vi "子界面-评定报告生成.vi"(1 "反射图路径":path, 5 "标注后的图片路径":path, 6 "总面积":i32, 7 "部位":string, 8 "穿透图路径":path, 9 "测试人":string, 10 "产品序号":string) -> (3 "写入数据库路径":path)   [LabVIEW 2018]
uses:
  <vilib>/Utility/NIReport.llb/Report Type.ctl
  <vilib>/addons/database/Connection.llb/DB Tools Open Connec (String).vi
  <vilib>/Utility/NIReport.llb/Append Report Text (str wrap).vi
  <vilib>/Utility/NIReport.llb/Append Report Text (num wrap).vi
  <vilib>/Utility/NIReport.llb/Append Image to Report (path wrap).vi
  <vilib>/addons/database/_DB Variant To Data/Database Variant To Data.xnode
  <vilib>/Utility/NIReport.llb/NI_report.lvclass
  <vilib>/addons/database/NI_Database_API.lvlib
  <vilib>/Utility/NIReport.llb/NI_ReportGenerationCore.lvlib
  <vilib>/Utility/NIReport.llb/Word/NI_Word.lvclass
panel:
  out "报告生成路径":path
  out "最大Z值":cluster{dbl}
  out "评定等级":string
  out "data":T1
  out "评定等级2":string caption="评定等级"
  out "缺陷占比(%)":dbl
  out "数值":dbl
  in  "返回 2":bool
  out "data 2":T1
  # "评定和分级结果"
  # "分层类"
  # "弥散类"
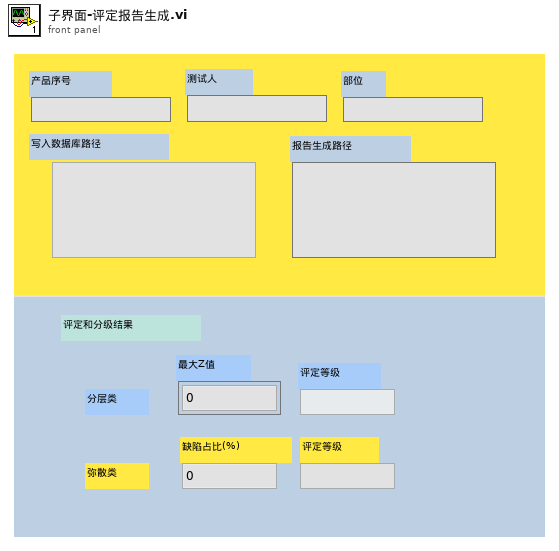
[diagram p1: front panel]
types:
  T1 = typedef "Z值ctl.ctl" = cluster{dbl}[]
  T2 = cluster{"position (excel)":cluster{"row":i32, "column":i32}, "name (excel)":string, "bookmark (word)":string}
  T3 = cluster{"position (Excel)":cluster{"row":i32, "column":i32}, "name (Excel)":string, "bookmark (Word)":string}
  T4 = typedef "NI_ReportGenerationCore.lvlib/Report Type.ctl" = enum16{"HTML", "Word", "Excel"}
  T5 = typedef "NI_Database_API.lvlib/Conn ObjectReference.ctl" = refnum<k1>
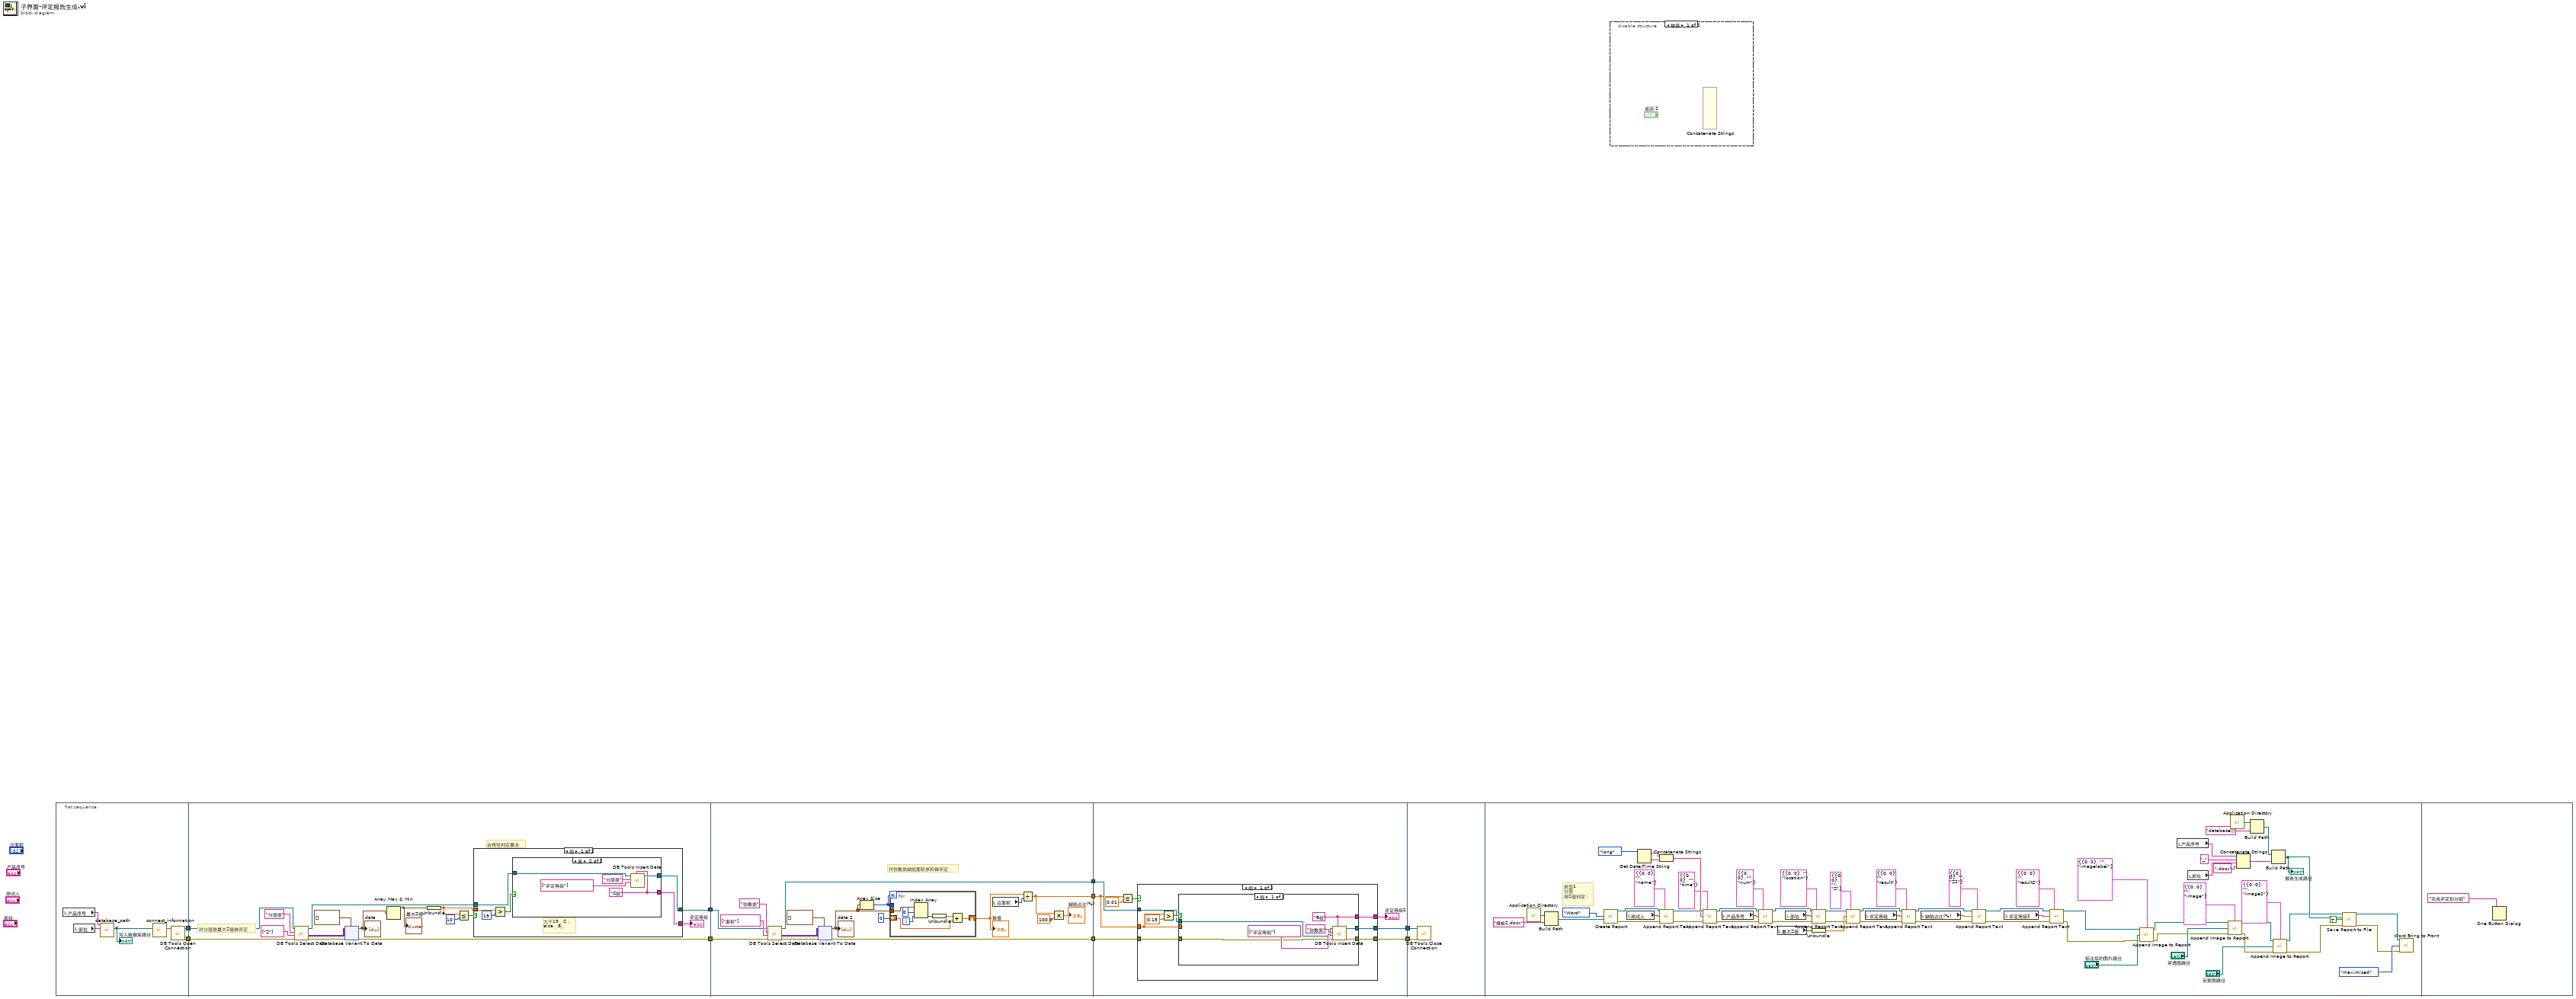
[diagram p0: block diagram]
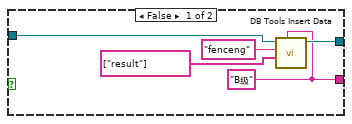
[diagram p2: hidden frame]
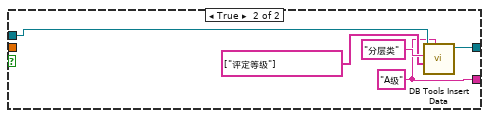
[diagram p3: hidden frame]
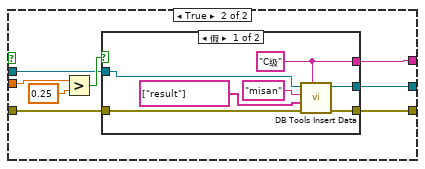
[diagram p4: hidden frame]
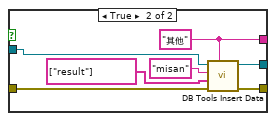
[diagram p5: hidden frame]
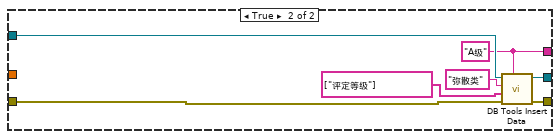
[diagram p6: hidden frame]
diagram:
  n1 = flat-sequence {
    tunnel: [w11] -> w9
    tunnel: [w10] -> w8
    tunnel: w9 -> [w25]
    tunnel: w8 -> [w28]
    tunnel: [w19] -> w7
    tunnel: [w17] -> w6
    tunnel: [w104] -> w5
    tunnel: w7 -> [w108]
    tunnel: w6 -> [w105]
    tunnel: [w103] -> w4
    tunnel: [w96] -> w3
    tunnel: w5 -> [w162]
    tunnel: w4 -> [w164]
    tunnel: [w163] -> w2
    tunnel: [w161] -> w1
    tunnel: w3 -> [w160]
    tunnel: w2 -> [w212]
    tunnel: w1 -> [w211]
    frame #0 {
      n2 = local read "产品序号"() -> (w13:string)
      n3 = local read "部位"() -> (w12:string)
      n4 = call "database_path.vi"("部位"=w12, "产品序号"=w13) -> ("database path"=w14:path)  [unwired: 9 in]
      "写入数据库路径" <- w14
      n5 = call "connect_information.vi"("路径"=w14) -> ("connect info"=w15:string)  [unwired: 10 in]
      n6 = call-poly <vilib>:"DB Tools Open Connection.vi"("connection information"=w15) -> ("error out"=w10:errorcluster, "connection reference"=w11:T5)  [unwired: 7 in]
    }
    frame #1 {
      # "合格性判定算法"
      # "对分层类最大Z值做评定"
      n7 = call <vilib>:"DB Tools Select Data.vi"("error in (no error)"=w28, "columns"=string[] ["Z"], "table"="分层类", "connection reference"=w25) -> ("error out"=w29:errorcluster, "data"=w27:variant[][], "connection reference out"=w20:T5)  [unwired: 2 in]
      n8 = xnode "Database Variant To Data"("database variant"=w27, "error in (no error)"=w29, "type"=T1 []) -> ("data"=w24:T1, "error out"=w17:errorcluster)
      "data" <- w24
      n9 = Array Max & Min(array=w24) -> (max value=w21:cluster{dbl})  [unwired: 3 out]
      "最大Z值" <- w21
      n10 = Unbundle(w21) -> (w18:dbl)
      n11 = Less Or Equal?(x=w18, y=10) -> (x <= y?=w22:bool)
      n12 = case shown="假" w22 {
        tunnel: w20 -> [w35 w52]
        tunnel: [w34 w49] -> w19
        tunnel: w18 -> [w33 _]
        tunnel: [w32 w48] -> w16
        frame False {
          # "大于19，C；\nelse，B。"
          n13 = Greater?(x=w33, y=19) -> (0:w36:bool)
          n14 = case shown="真" w36 {
            tunnel: w35 -> [w40 w44]
            tunnel: [w39 w45] -> w34
            tunnel: [w38 w43] -> w32
            frame False {
              w38 = "B级"
              n15 = call <vilib>:"DB Tools Insert Data.vi"("data"=w38, "columns"=string[] ["result"], "table"="fenceng", "connection reference"=w40) -> ("connection reference out"=w39:T5)  [unwired: 6 in, 1 out]
            }
            frame True {
              w43 = "C级"
              n16 = call <vilib>:"DB Tools Insert Data.vi"("data"=w43, "columns"=string[] ["评定等级"], "table"="分层类", "connection reference"=w44) -> ("connection reference out"=w45:T5)  [unwired: 6 in, 1 out]
            }
          }
        }
        frame True {
          w48 = "A级"
          n17 = call <vilib>:"DB Tools Insert Data.vi"("data"=w48, "columns"=string[] ["评定等级"], "table"="分层类", "connection reference"=w52) -> ("connection reference out"=w49:T5)  [unwired: 6 in, 1 out]
        }
      }
      "评定等级" <- w16
    }
    frame #2 {
      # "对弥散类缺陷面积求和做评定"
      n18 = call <vilib>:"DB Tools Select Data.vi"("error in (no error)"=w105, "columns"=string[] ["面积"], "table"="弥散类", "connection reference"=w108) -> ("error out"=w106:errorcluster, "data"=w107:variant[][], "connection reference out"=w103:T5)  [unwired: 2 in]
      n19 = xnode "Database Variant To Data"("database variant"=w107, "error in (no error)"=w106, "type"=T1 []) -> ("data"=w101:T1, "error out"=w104:errorcluster)
      "data 2" <- w101
      n20 = Array Size(array=w101) -> (size(s)=w100:i32)
      n21 = for {
        N: w100 -> [_]
        tunnel: w101 -> [w117]
        tunnel: w100 -> [_]
        shift-right: [w112] -> w98
        shift-left: 0 -> [w111]
        i -> [w115]
        n22 = Index Array(array=w117, index #1=0 ("索引 (列)"), index #2=w115) -> (element #2=w114:cluster{dbl})  [unwired: 1 out]
        n23 = Unbundle(w114) -> (w113:dbl)
        n24 = Add(x=w113, y=w111) -> (x+y=w112:dbl)
      }
      "数值" <- w98
      n25 = local read "总面积"() -> (w97:i32)
      n26 = Divide(x=w98, y=w97) -> (x/y=w96:dbl)
      n27 = Multiply(x=w96, y=100.0) -> (x*y=→"缺陷占比(%)":dbl)
    }
    frame #3 {
      n28 = Less Or Equal?(x=w160, y=0.01) -> (x <= y?=w166:bool)
      n29 = case shown="假" w166 {
        tunnel: w164 -> [w171 w208]
        tunnel: [w170 w207] -> w163
        tunnel: w162 -> [w168 w206]
        tunnel: [w169 w205] -> w161
        tunnel: w160 -> [w172 _]
        tunnel: [w167 w204] -> w159
        frame False {
          n30 = Greater?(x=w172, y=0.15) -> (0:w173:bool)
          n31 = case shown="假" w173 {
            tunnel: w172 -> [_ w187]
            tunnel: w171 -> [w179 w186]
            tunnel: [w178 w185] -> w170
            tunnel: [w177 w184] -> w169
            tunnel: w168 -> [w176 w183]
            tunnel: [w175 w182] -> w167
            frame False {
              w175 = "B级"
              n32 = call <vilib>:"DB Tools Insert Data.vi"("data"=w175, "error in (no error)"=w176, "columns"=string[] ["评定等级"], "table"="弥散类", "connection reference"=w179) -> ("error out"=w177:errorcluster, "connection reference out"=w178:T5)  [unwired: 5 in]
            }
            frame True {
              n33 = Greater?(x=w187, y=0.25) -> (0:w188:bool)
              n34 = case shown="假" w188 {
                tunnel: w186 -> [w194 w201]
                tunnel: [w193 w200] -> w185
                tunnel: [w192 w199] -> w184
                tunnel: w183 -> [w191 w198]
                tunnel: [w190 w197] -> w182
                frame False {
                  w190 = "C级"
                  n35 = call <vilib>:"DB Tools Insert Data.vi"("data"=w190, "error in (no error)"=w191, "columns"=string[] ["result"], "table"="misan", "connection reference"=w194) -> ("error out"=w192:errorcluster, "connection reference out"=w193:T5)  [unwired: 5 in]
                }
                frame True {
                  w197 = "其他"
                  n36 = call <vilib>:"DB Tools Insert Data.vi"("data"=w197, "error in (no error)"=w198, "columns"=string[] ["result"], "table"="misan", "connection reference"=w201) -> ("error out"=w199:errorcluster, "connection reference out"=w200:T5)  [unwired: 5 in]
                }
              }
            }
          }
        }
        frame True {
          w204 = "A级"
          n37 = call <vilib>:"DB Tools Insert Data.vi"("data"=w204, "error in (no error)"=w206, "columns"=string[] ["评定等级"], "table"="弥散类", "connection reference"=w208) -> ("error out"=w205:errorcluster, "connection reference out"=w207:T5)  [unwired: 5 in]
        }
      }
      "评定等级2" <- w159
    }
    frame #4 {
      n38 = call <vilib>:"DB Tools Close Connection.vi"("error in (no error)"=w211, "connection reference"=w212) -> ()  [unwired: 5 in, 1 out]
    }
    frame #5 {
      # "类型1\n分层\n用Z值判定："
      n39 = call <vilib>:"Application Directory.vi"() -> ("Application Directory"=w279:path)
      n40 = Build Path(base path=w279, name or relative path="模板2.docx") -> (appended path=w278:path)
      n41 = call <vilib>:"Create Report.vi"("report type"=Report_Type."Word" ("Report Type"), "template (empty)"=w278) -> ("report out"=w261:refnum<class "NI_report.lvclass">, "error out"=w260:errorcluster)  [unwired: 12 in]
      n42 = local read "测试人"() -> (w259:string)
      n43 = Get Date/Time String(date format (0)=enum16{"short", "long", "abbreviated"}."long" ("日期格式(0)")) -> (date string=w267:string, time string=w269:string)  [unwired: 2 in]
      n44 = Concatenate Strings(w267, w269) -> (w268:string)
      n45 = call-poly <vilib>:"Append Report Text.vi"("report in"=w261, "MS Office parameters"=T3 {"position (Excel)"={"row"=0, "column"=0}, "name (Excel)"="", "bookmark (Word)"="name"}, "text"=w259, "error in (no error)"=w260) -> ("report out"=w272:refnum<class "NI_report.lvclass">, "error out"=w273:errorcluster)  [unwired: 8 in, 2 out]
      n46 = call-poly <vilib>:"Append Report Text.vi"("report in"=w272, "MS Office parameters"=T3 {"position (Excel)"={"row"=0, "column"=0}, "name (Excel)"="", "bookmark (Word)"="time"}, "text"=w268, "error in (no error)"=w273) -> ("report out"=w270:refnum<class "NI_report.lvclass">, "error out"=w271:errorcluster)  [unwired: 8 in, 2 out]
      n47 = local read "产品序号"() -> (w258:string)
      n48 = call-poly <vilib>:"Append Report Text.vi"("report in"=w270, "MS Office parameters"=T3 {"position (Excel)"={"row"=0, "column"=0}, "name (Excel)"="", "bookmark (Word)"="num"}, "text"=w258, "error in (no error)"=w271) -> ("report out"=w274:refnum<class "NI_report.lvclass">, "error out"=w275:errorcluster)  [unwired: 8 in, 2 out]
      n49 = local read "最大Z值"() -> (w251:cluster{dbl})
      n50 = local read "部位"() -> (w257:string)
      n51 = call-poly <vilib>:"Append Report Text.vi"("report in"=w274, "MS Office parameters"=T3 {"position (Excel)"={"row"=0, "column"=0}, "name (Excel)"="", "bookmark (Word)"="location"}, "text"=w257, "error in (no error)"=w275) -> ("report out"=w247:refnum<class "NI_report.lvclass">, "error out"=w246:errorcluster)  [unwired: 8 in, 2 out]
      n52 = Unbundle(w251) -> (w252:dbl)
      n53 = call-poly <vilib>:"Append Report Text.vi"("report in"=w247, "MS Office parameters"=T3 {"position (Excel)"={"row"=0, "column"=0}, "name (Excel)"="", "bookmark (Word)"="Z"}, "text"=w252, "error in (no error)"=w246) -> ("report out"=w245:refnum<class "NI_report.lvclass">, "error out"=w244:errorcluster)  [unwired: 8 in, 2 out]
      n54 = local read "评定等级"() -> (w250:string)
      n55 = call-poly <vilib>:"Append Report Text.vi"("report in"=w245, "MS Office parameters"=T3 {"position (Excel)"={"row"=0, "column"=0}, "name (Excel)"="", "bookmark (Word)"="result"}, "text"=w250, "error in (no error)"=w244) -> ("report out"=w243:refnum<class "NI_report.lvclass">, "error out"=w242:errorcluster)  [unwired: 8 in, 2 out]
      n56 = local read "缺陷占比(%)"() -> (w249:dbl)
      n57 = call-poly <vilib>:"Append Report Text.vi"("report in"=w243, "MS Office parameters"=T3 {"position (Excel)"={"row"=0, "column"=0}, "name (Excel)"="", "bookmark (Word)"="Z2"}, "text"=w249, "error in (no error)"=w242) -> ("report out"=w241:refnum<class "NI_report.lvclass">, "error out"=w240:errorcluster)  [unwired: 8 in, 2 out]
      n58 = local read "评定等级2"() -> (w248:string)
      n59 = call-poly <vilib>:"Append Report Text.vi"("report in"=w241, "MS Office parameters"=T3 {"position (Excel)"={"row"=0, "column"=0}, "name (Excel)"="", "bookmark (Word)"="result2"}, "text"=w248, "error in (no error)"=w240) -> ("report out"=w216:refnum<class "NI_report.lvclass">, "error out"=w214:errorcluster)  [unwired: 8 in, 2 out]
      n60 = call-poly <vilib>:"Append Image to Report.vi"("report in"=w216, "MS Office parameters"=T2 {"position (excel)"={"row"=0, "column"=0}, "name (excel)"="", "bookmark (word)"="imagelabel"}, "path or URL of image"="标注后的图片路径", "error in (no error)"=w214) -> ("report out"=w215:refnum<class "NI_report.lvclass">, "error out"=w213:errorcluster)  [unwired: 8 in, 2 out]
      n61 = local read "产品序号"() -> (w235:string)
      n62 = local read "部位"() -> (w234:string)
      n63 = call-poly <vilib>:"Append Image to Report.vi"("report in"=w215, "MS Office parameters"=T3 {"position (Excel)"={"row"=0, "column"=0}, "name (Excel)"="", "bookmark (Word)"="image"}, "path or URL of image"="穿透图路径", "error in (no error)"=w213) -> ("report out"=w228:refnum<class "NI_report.lvclass">, "error out"=w221:errorcluster)  [unwired: 8 in, 2 out]
      n64 = call <vilib>:"Application Directory.vi"() -> ("Application Directory"=w232:path)
      n65 = Concatenate Strings(w235, "_" ("名称或相对路径"), w234, ".docx" ("名称或相对路径")) -> (w238:string)
      n66 = Build Path(base path=w232, name or relative path="database\\" ("名称或相对路径")) -> (appended path=w230:path)
      n67 = Build Path(base path=w230, name or relative path=w238) -> (appended path=w233:path)
      "报告生成路径" <- w233
      n68 = call-poly <vilib>:"Append Image to Report.vi"("report in"=w228, "MS Office parameters"=T3 {"position (Excel)"={"row"=0, "column"=0}, "name (Excel)"="", "bookmark (Word)"="image2"}, "path or URL of image"="反射图路径", "error in (no error)"=w221) -> ("report out"=w226:refnum<class "NI_report.lvclass">, "error out"=w222:errorcluster)  [unwired: 8 in, 2 out]
      n69 = call-dynamic "Save Report to File.vi"("report in"=w226, "report file path"=w233, "prompt to replace? (F)"=TRUE, "error in (no error)"=w222) -> ("report out"=w224:refnum<class "NI_report.lvclass">, "error out"=w223:errorcluster)  [unwired: 10 in]
      n70 = call <vilib>:"Word Bring to Front.vi"("report in"=w224, "window state (maximized)"=enum16{"maximized", "minimized", "normal"}."maximized", "error in (no error)"=w223) -> ()  [unwired: 11 in, 2 out]
    }
    frame #6 {
      n71 = One Button Dialog(message="完成评定和分级" ("消息")) -> ()  [unwired: 1 in, 1 out]
    }
  }
  n72 = disable-structure shown="禁用" {
    frame Disabled {
      n73 = Concatenate Strings() -> ()  [unwired: 12 in, 1 out]
    }
    frame Enabled {
    }
  }
